vi "Banana_Not Equal Type Comparison.vi"(8 "error in (no error)":errorcluster, 9 "Y":variant, 10 "X":variant) -> (0 "error out":errorcluster, 2 "Not Equal Types?":bool)   [LabVIEW 2021, in "Bananas.lvlib"]
uses:
  Bananas.lvlib
  <vilib>/Utility/Data Type/NI_Data Type.lvlib
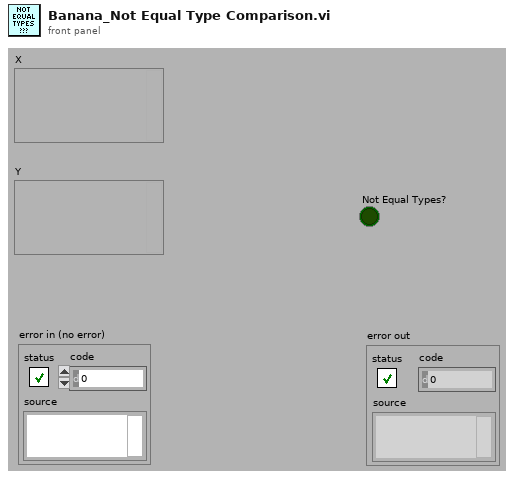
[diagram p1: front panel]
types:
  T1 = typedef "NI_Data Type.lvlib/Data Type.ctl" = enum8{"Invalid Type", "Void", "I8", "I16", "I32", "I64", "U8", "U16", "U32", "U64", "Single Float", "Double Float", "Extended Float", "Single Complex", "Double Complex", "Extended Complex", "Enum U8", "Enum U16", "Enum U32", "Enum U64", "Single Float With Unit", "Double Float With Unit", "Extended Float With Unit", "Single Complex with Unit", "Double Complex with Unit", "Extended Complex with Unit", "Boolean", "String", "Path", "Picture", "Tag", "Array", "Cluster", "Variant", "LV Variant", "Waveform", "Timestamp", "Digital Waveform", "Digital Data", "ExpressData", "Refnum", "External Data", "VI", "Poly VI", "LabVIEW Class Instance", "Fixed Point", "Set Collection", "Map Collection"}
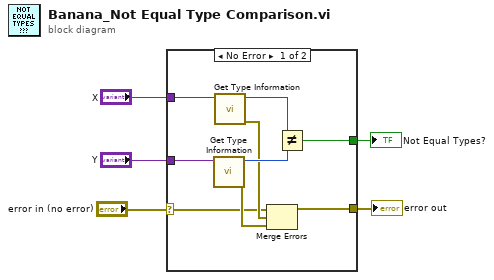
[diagram p0: block diagram]
diagram:
  n1 = case shown="No Error" "error in (no error)" {
    selector: "error in (no error)" -> [w6 w15]
    tunnel: "X" -> [w12 _]
    tunnel: "Y" -> [w10 _]
    tunnel: [w14 w15] -> w5
    tunnel: [w13 _] -> w4
    frame No Error {
      n2 = call <vilib>:"Get Type Information.vi"("variant"=w10) -> ("error out"=w7:errorcluster, "type"=w9:T1)  [unwired: 6 in, 3 out]
      n3 = call <vilib>:"Get Type Information.vi"("variant"=w12) -> ("error out"=w8:errorcluster, "type"=w11:T1)  [unwired: 6 in, 3 out]
      n4 = Merge Errors(w6, w8, w7) -> (w14:errorcluster)
      n5 = Not Equal?(x=w11, y=w9) -> (x != y?=w13:bool)
    }
    frame Error {
    }
  }
  "Not Equal Types?" <- w4
  "error out" <- w5
